vi "VI Server_MenuRing_U16_Selection_Get.vi"(7 "Control.Label":string, 8 "error in":errorcluster, 9 "SingleInstance":bool, 11 "VI Server.Cluster":T1) -> (0 "error out":errorcluster, 1 "Control.Ref":refnum<vi>, 2 "M-Ring.Selection":string, 3 "VI Server.Cluster.DUP":T1)   [LabVIEW 2020]
uses:
  VI Server_TypeDefs/VI Server_RefsCluster.ctl
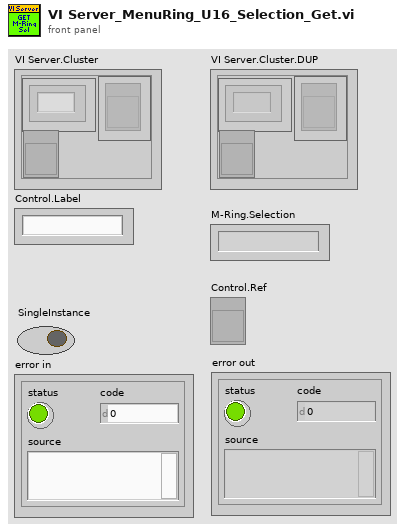
[diagram p1: front panel]
types:
  T1 = typedef "VI Server_RefsCluster.ctl" = cluster{"Labels":string[], "Refs":refnum<vi>[], "VI Ref":refnum<vi>}
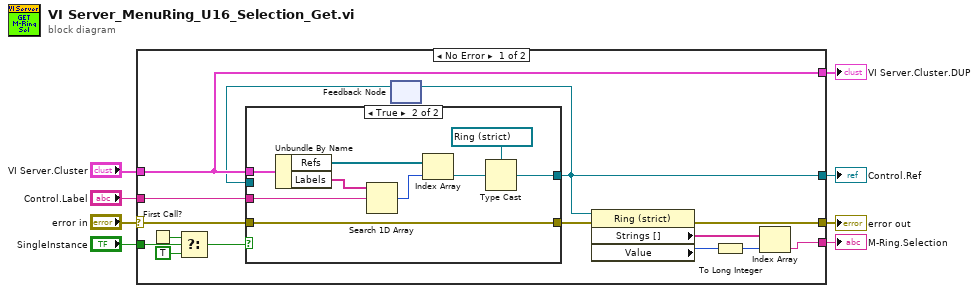
[diagram p0: block diagram]
diagram:
  n1 = case shown="No Error" "error in" {
    selector: "error in" -> [w22 w35]
    tunnel: "VI Server.Cluster" -> [w21 _]
    tunnel: "Control.Label" -> [w23 _]
    tunnel: [w15 w35] -> w5
    tunnel: [w13 _] -> w2
    tunnel: [w21 _] -> w4
    tunnel: "SingleInstance" -> [w20 _]
    tunnel: [w10 _] -> w1
    frame No Error {
      n2 = First Call?() -> (First Call?: T/F=w18:bool)
      n3 = Select(t=w18, s=w20, f=TRUE) -> (s? t:f=w19:bool)
      n4 = feedback #1() -> (w16:refnum<vi>)  [unwired: 1 in]
      n5 = case shown="True" w19 {
        tunnel: w23 -> [_ w33]
        tunnel: w22 -> [w24 w29]
        tunnel: [w24 w29] -> w14
        tunnel: [w25 w27] -> w13
        tunnel: w21 -> [_ w28]
        tunnel: w16 -> [w25 _]
        frame False {
        }
        frame True {
          n6 = Unbundle By Name(w28) -> ("Refs"=w32:refnum<vi>[], "Labels"=w34:string[])
          n7 = Search 1D Array(1D array=w34, element=w33) -> (index of element=w31:i32)  [unwired: 1 in]
          n8 = Index Array(array=w32, index=w31) -> (element=w30:refnum<vi>)
          n9 = Type Cast(type=refnum<vi> refnum ("DataType"), x=w30) -> (*(type *) &x=w27:refnum<vi>)
        }
      }
      n10 = feedback-in #1(w13) -> ()
      n11 = property class="Ring (strict)"(reference=w13, error in=w14) -> (error out=w15:errorcluster, "Strings []"=w12:string[], "Value"=w11:u16)  [unwired: 1 out]
      n12 = To Long Integer(number=w11) -> (32bit integer=w9:i32)
      n13 = Index Array(array=w12, index=w9) -> (element=w10:string)
    }
    frame Error {
    }
  }
  "VI Server.Cluster.DUP" <- w4
  "error out" <- w5
  "M-Ring.Selection" <- w1
  "Control.Ref" <- w2
